vi "Cleanup.vi"(8 "error in (no error)":errorcluster, 11 "LV Server in":refnum<class "LV Server.lvclass">) -> (0 "error out":errorcluster)   [LabVIEW 2020, in "LV Server.lvclass"]
uses:
  LV Server.lvclass
  LV Server.lvclass/LV Server.ctl
  <vilib>/IlluminatedG/lv-msg-simple/Stream-Simple-Msg/Manager/Manager.lvclass
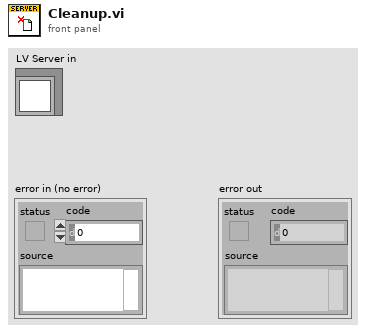
[diagram p1: front panel]
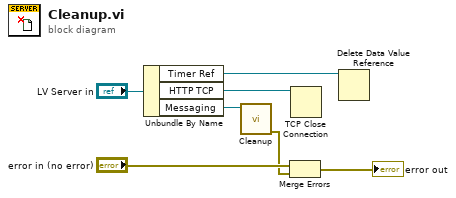
[diagram p0: block diagram]
diagram:
  n1 = Unbundle By Name("LV Server in") -> ("Timer Ref"=w4:refnum<data-value>, "HTTP TCP"=w5:refnum<k5>, "Messaging"=w3:refnum<class "Manager.lvclass">)
  n2 = call <vilib>:"Cleanup.vi"("Manager in"=w3) -> ("error out"=w1:errorcluster)  [unwired: 10 in]
  n3 = Merge Errors("error in (no error)", w1) -> (→"error out":errorcluster)
  n4 = TCP Close Connection(connection ID=w5) -> ()  [unwired: 2 in, 2 out]
  n5 = Delete Data Value Reference(data value reference=w4) -> ()  [unwired: 1 in, 2 out]
